vi "Get Data Word Format.vi"(8 "error in":errorcluster, 11 "logging in":T2=18446744073709551615 format="%.0x") -> (0 "error out":errorcluster, 2 "data word format":T1, 3 "logging out":T2 format="%.0x")   [LabVIEW 2020, in "AIM MIL-STD-1553 Scripting.lvlib"]
doc: "Returns the format of data words in the log file."
uses:
  AIM MIL-STD-1553 Scripting.lvlib
  <vilib>/NI VeriStand/Custom Device API/Custom Device Item Ref.ctl
  Shared/Data Word Format.ctl
  Constants.vi
  <vilib>/NI VeriStand/Custom Device API/Get Item Property (String).vi
  <vilib>/NI VeriStand/Custom Device API/Custom Device API.lvlib
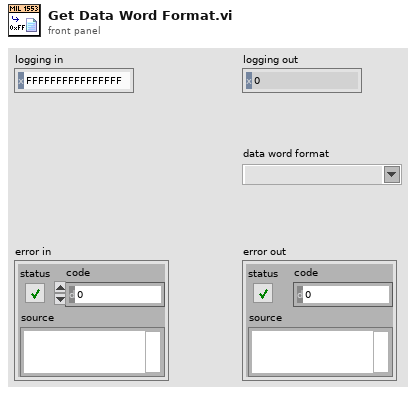
[diagram p1: front panel]
types:
  T1 = typedef "Data Word Format.ctl" = string
  T2 = typedef "Custom Device API.lvlib/Custom Device Item Ref.ctl" = u64
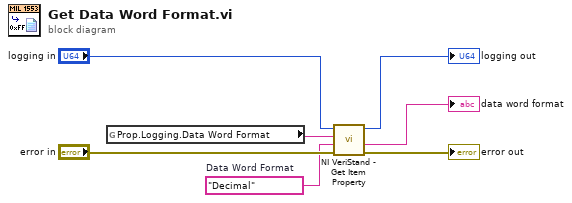
[diagram p0: block diagram]
diagram:
  w2 = T1 "Decimal"  # Data Word Format
  n1 = global read "Constants.vi" "Prop.Logging.Data Word Format"() -> (w1:string)
  n2 = call-poly <vilib>:"NI VeriStand - Get Item Property.vi"("error in (no error)"="error in", "Default Value"=w2, "Property Name"=w1, "Item Ref in"="logging in") -> ("error out"=→"error out":errorcluster, "Value"=→"data word format":string, "Item Ref out"=→"logging out":T2)  [unwired: 4 in, 1 out]
